vi "Get BuildWorker Name.vi"(8 "error in (no error)":errorcluster, 11 "BuildWorker Controller in":refnum<class "BuildWorker Controller.lvclass">) -> (0 "error out":errorcluster, 2 "Name":string, 3 "BuildWorker Controller out":refnum<class "BuildWorker Controller.lvclass">)   [LabVIEW 2017, in "BuildWorker Controller.lvclass"]
uses:
  BuildWorker Controller.lvclass
  BuildWorker Controller.lvclass/BuildWorker Controller.ctl
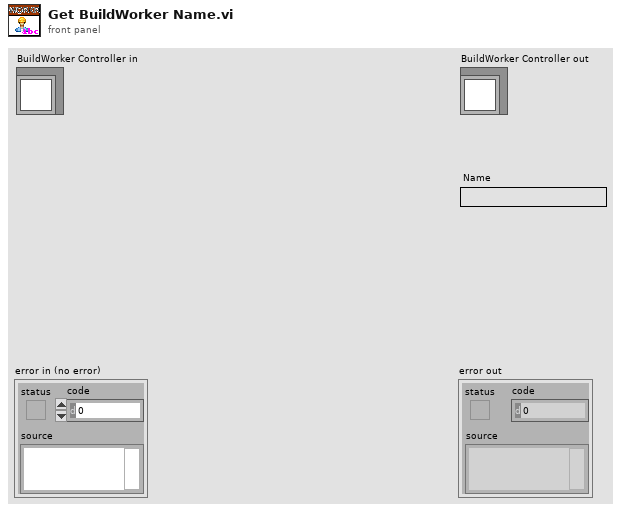
[diagram p1: front panel]
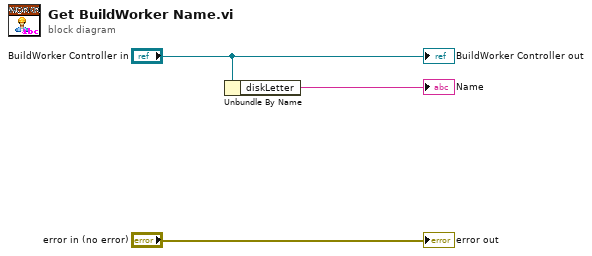
[diagram p0: block diagram]
diagram:
  n1 = Unbundle By Name("BuildWorker Controller in") -> ("diskLetter"=→"Name":string)
  "error out" <- "error in (no error)"
  "BuildWorker Controller out" <- "BuildWorker Controller in"
